vi "set_instruments (SubVI).vi"(1 "set_instrument inputs":T2={"wfm?"=FALSE, "User Def. Wfm Name"="RANDFREQ", "Enable Output?"=TRUE, "Trigger Synth"=FALSE, "Burst Count"=1, "Arbitrary Waveform Data"=[]}, 2 "keysight":bool, 4 "Chan 2":bool, 6 "time":dbl, 7 "change?":bool, 8 "Process list":T5, 9 "initialized output":T1, 10 "flip iteration":i16, 11 "Flash lamp settings:":T4={"Output channel (for flashing)"="Dev4/ao0", "Loop iteration"=0, "Path"=path "", "Flash lamp\n settings:"={"Flash lamp?"=FALSE, "Number of cyles\nbetween flashes"=3, "# Pulses"=35, "Stop flashing \nbelow thresh?"=FALSE, "Stop threshold"=0.001, "Pulse amp (V)"=0.001}}) -> (0 "instrum out":T3, 3 "Curr threshold":dbl, 5 "Axes position":i32[](array[numeric]))   [LabVIEW 2018]
uses:
  C:/Users/yalem/GitHub/Documents/Optlev/LabView Code/Examples/Tilt Stage/CmdLib.dll
  Examples/Tilt Stage/CmdLib.dll
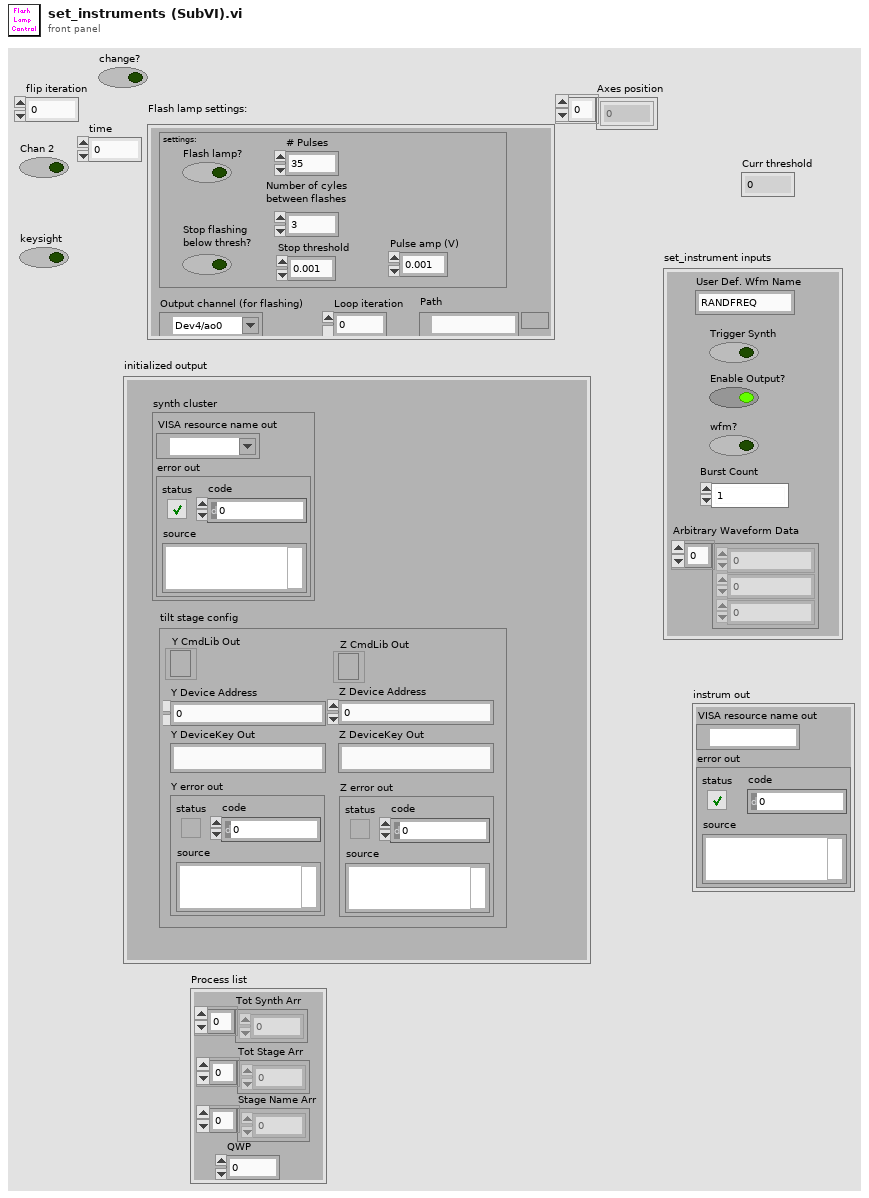
[diagram p1: front panel]
types:
  T1 = cluster{"synth cluster":cluster{"VISA resource name out":refnum<visa-resource-name>, "error out":errorcluster}, "tilt stage config":cluster{"Y error out":errorcluster, "Y CmdLib Out":refnum<k24>, "Y Device Address":i32, "Y DeviceKey Out":string, "Z error out":errorcluster, "Z CmdLib Out":refnum<k24>, "Z Device Address":i32, "Z DeviceKey Out":string}}
  T2 = cluster{"wfm?":bool, "User Def. Wfm Name":string, "Enable Output?":bool, "Trigger Synth":bool, "Burst Count":i32, "Arbitrary Waveform Data":dbl[]}
  T3 = cluster{"VISA resource name out":refnum<visa-resource-name>, "error out":errorcluster}
  T4 = cluster{"Output channel (for flashing)":tag, "Loop iteration":i32, "Path":path, "Flash lamp\n settings:":cluster{"Flash lamp?":bool, "Number of cyles\nbetween flashes":i32, "# Pulses":i32, "Stop flashing \nbelow thresh?":bool, "Stop threshold":dbl, "Pulse amp (V)":dbl}}
  T5 = cluster{"Tot Synth Arr":dbl[], "Tot Stage Arr":dbl[], "Stage Name Arr":dbl[], "QWP":dbl}
  T6 = cluster{"Flash lamp?":bool, "Number of cyles\nbetween flashes":i32, "# Pulses":i32, "Stop flashing \nbelow thresh?":bool, "Stop threshold":dbl, "Pulse amp (V)":dbl}
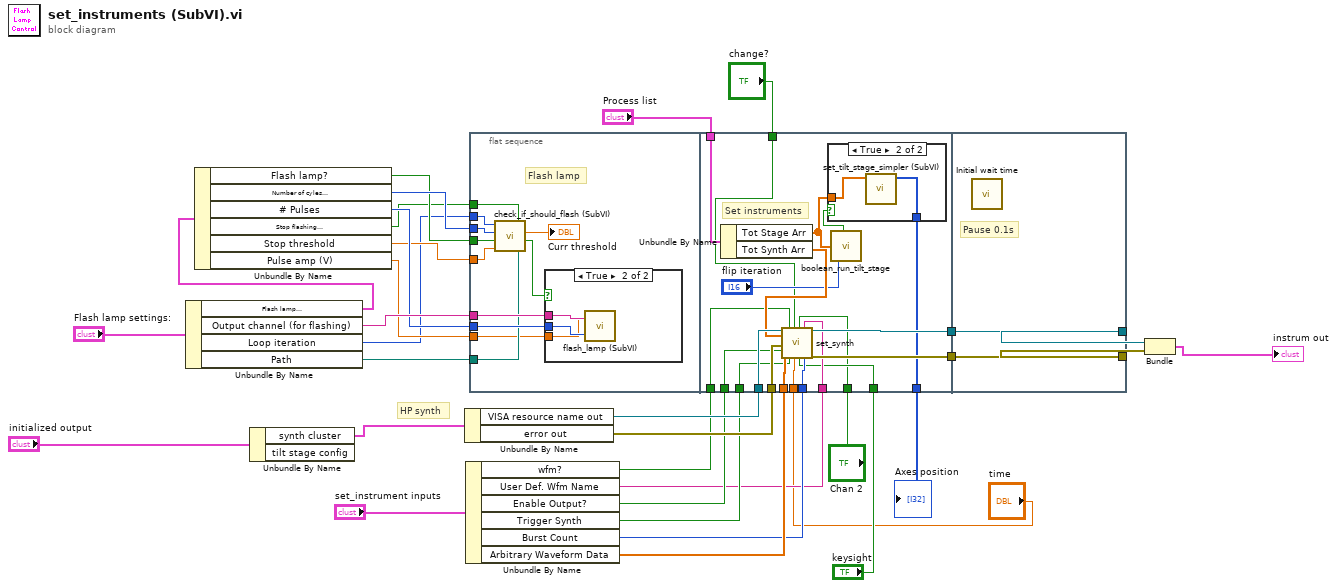
[diagram p0: block diagram]
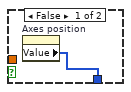
[diagram p3: hidden frame]
diagram:
  # "HP synth"
  n1 = Unbundle By Name("Flash lamp settings:") -> ("Flash lamp\n settings:"=w20:T6, "Output channel (for flashing)"=w31:tag, "Loop iteration"=w7:i32, "Path"=w27:path)
  n2 = Unbundle By Name(w20) -> ("Flash lamp?"=w28:bool, "Number of cyles\nbetween flashes"=w29:i32, "# Pulses"=w30:i32, "Stop flashing \nbelow thresh?"=w25:bool, "Stop threshold"=w26:dbl, "Pulse amp (V)"=w19:dbl)
  n3 = Unbundle By Name("initialized output") -> ("synth cluster"=w17:T3)  [unwired: 1 out]
  n4 = Unbundle By Name(w17) -> ("VISA resource name out"=w24:refnum<visa-resource-name>, "error out"=w23:errorcluster)
  n5 = Unbundle By Name("set_instrument inputs") -> ("wfm?"=w10:bool, "User Def. Wfm Name"=w11:string, "Enable Output?"=w12:bool, "Trigger Synth"=w13:bool, "Burst Count"=w14:i32, "Arbitrary Waveform Data"=w15:dbl[])
  n6 = flat-sequence {
    tunnel: w31 -> [w44]
    tunnel: w30 -> [w43]
    tunnel: w7 -> [w42]
    tunnel: w29 -> [w41]
    tunnel: w28 -> [w40]
    tunnel: w27 -> [w39]
    tunnel: w26 -> [w38]
    tunnel: w25 -> [w34]
    tunnel: w19 -> [w36]
    tunnel: "Process list" -> [w67]
    tunnel: w24 -> [w66]
    tunnel: w23 -> [w65]
    tunnel: [w63] -> w9
    tunnel: [w64] -> w8
    tunnel: w15 -> [w59]
    tunnel: w14 -> [w58]
    tunnel: w13 -> [w57]
    tunnel: w12 -> [w56]
    tunnel: w11 -> [w55]
    tunnel: w10 -> [w54]
    tunnel: [w52] -> w6
    tunnel: "keysight" -> [w51]
    tunnel: "Chan 2" -> [w50]
    tunnel: "change?" -> [w49]
    tunnel: "time" -> [w48]
    tunnel: [w71] -> w21
    tunnel: [w72] -> w22
    tunnel: w9 -> [w72]
    tunnel: w8 -> [w71]
    frame #0 {
      # "Flash lamp"
      n7 = call "check_if_should_flash (SubVI).vi"("Path"=w39, "Stop below threshold"=w34, "Stop threshold"=w38, "Flash lamp?"=w40, "Number of cyles\nbetween flashes"=w41, "Loop iteration"=w42) -> ("Should flash"=w35:bool, "Curr threshold"=→"Curr threshold":dbl)
      n8 = case shown="True" w35 {
        tunnel: w44 -> [_ w47]
        tunnel: w43 -> [_ w46]
        tunnel: w36 -> [_ w45]
        frame False {
        }
        frame True {
          n9 = call "flash_lamp (SubVI).vi"("Pulse amp (V)"=w45, "# Pulses in"=w46, "Output channel (for flashing)"=w47) -> ()  [unwired: 1 in]
        }
      }
    }
    frame #1 {
      # "Set instruments"
      n10 = Unbundle By Name(w67) -> ("Tot Stage Arr"=w61:dbl[], "Tot Synth Arr"=w62:dbl[])
      n11 = call "set_synth.vi"("VISA resource name"=w66, "Tot Synth Arr"=w62, "error in (no error)"=w65, "Enable Output (T: Enable)"=w56, "Arbitrary Waveform Data"=w59, "wfm?"=w54, "Trigger Synth"=w57, "change?"=w49, "time"=w48, "Chan 2"=w50, "keysight"=w51, "Arbitrary Waveform Name (\"ARB1\")"=w55, "Burst Count"=w58) -> ("VISA resource name out"=w63:refnum<visa-resource-name>, "error out"=w64:errorcluster)  [unwired: 5 in]
      n12 = call "boolean_run_tilt_stage.vi"("flip iteration"="flip iteration", "Tot Stage Arr"=w61) -> ("run tilt stage"=w60:bool)  [unwired: 1 in]
      n13 = case shown="True" w60 {
        tunnel: w61 -> [_ w70]
        tunnel: [w68 w69] -> w52
        frame False {
          n14 = property on="Axes position" class="Arr (strict)"() -> ("Value"=w68:i32[])  [unwired: 2 in, 2 out]
        }
        frame True {
          n15 = call "set_tilt_stage_simpler (SubVI).vi"("Tot Stage Arr"=w70) -> ("Axes position"=w69:i32[])  [unwired: 10 in]
        }
      }
    }
    frame #2 {
      # "Pause 0.1s"
      n16 = call "Initial wait time"() -> ()  [unwired: 11 in, 1 out]
    }
  }
  n17 = Bundle("VISA resource name out"=w22, "error out"=w21) -> (→"instrum out":T3)  [unwired: 1 in]
  "Axes position" <- w6
